vi "Update_TTL_IO_times-to-live.vi"(8 "error in (no error)":errorcluster, 10 "IO ports status in":T1, 11 "Previous loop time, us":i32) -> (0 "error out":errorcluster, 3 "IO ports status out":i32[][](array[numeric]))   [LabVIEW 2018, in "TTL IO.lvlib"]
uses:
  TTL IO.lvlib
  Typedefs/CTL_IO_ports_status.ctl
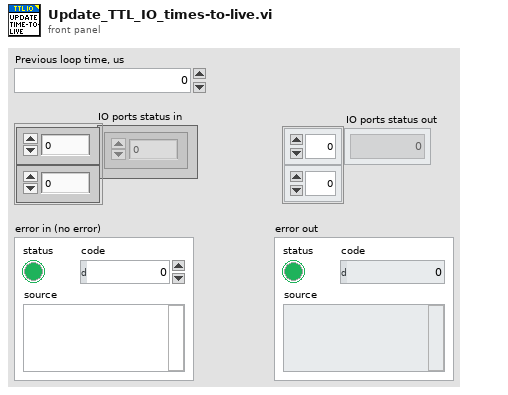
[diagram p1: front panel]
types:
  T1 = typedef "TTL IO.lvlib/CTL_IO_ports_status.ctl" = i32[][]
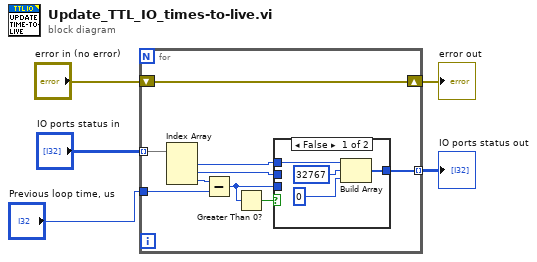
[diagram p0: block diagram]
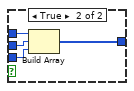
[diagram p2: hidden frame]
diagram:
  n1 = for {
    tunnel: "Previous loop time, us" -> [w12]
    shift-right: [w6] -> w5
    shift-left: "error in (no error)" -> [w6]
    tunnel: "IO ports status in" -> [w14] mode=indexing
    tunnel: [w7] -> w1 mode=indexing
    n2 = Index Array(array=w14) -> (element #1=w8:i32, element #2=w9:i32, element #3=w13:i32)  [unwired: 3 in]
    n3 = Subtract(x=w13, y=w12) -> (x-y=w10:i32)
    n4 = Greater Than 0?(x=w10) -> (x > 0?=w11:bool)
    n5 = case shown="False" w11 {
      tunnel: w10 -> [_ w20]
      tunnel: w9 -> [_ w21]
      tunnel: w8 -> [w18 w22]
      tunnel: [w15 w19] -> w7
      frame False {
        n6 = Build Array(w18, 32767 ("element"), 0 ("element")) -> (w15:i32[])
      }
      frame True {
        n7 = Build Array(w22, w21, w20) -> (w19:i32[])
      }
    }
  }
  "error out" <- w5
  "IO ports status out" <- w1
